vi "solar_read SOLARAppInfo.vi"(8 "error in (no error)":errorcluster, 11 "solar in":refnum<class "solar.lvclass">) -> (0 "error out":errorcluster, 2 "AppInfo":T1, 3 "solar out":refnum<class "solar.lvclass">)   [LabVIEW 2018, in "solar.lvclass"]
doc: "This returns the application information including application directories and versions information."
uses:
  solar.lvclass
  app/solar_app_ctl Info.ctl
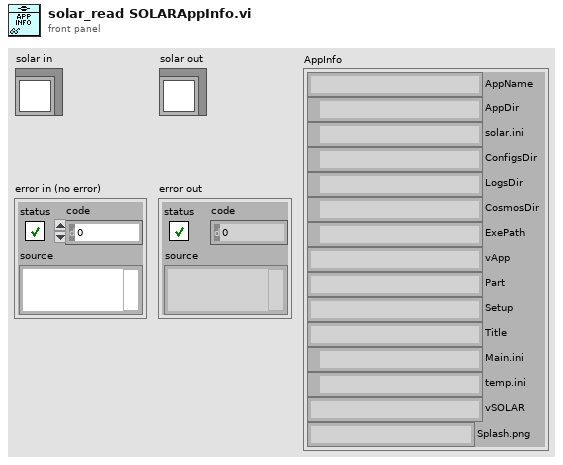
[diagram p1: front panel]
types:
  T1 = typedef "solar_app_ctl Info.ctl" = cluster{"AppName":string, "AppDir":path, "solar.ini":path, "ConfigsDir":path, "LogsDir":path, "CosmosDir":path, "ExePath":path, "vApp":string, "Part":string, "Setup":string, "Title":string, "Main.ini":path, "temp.ini":path, "vSOLAR":string, "Splash.png":string}
  T2 = typedef "solar_ctl SOLAR Refnum.ctl" = refnum<k1>
  T3 = typedef "solar_ctl SOLAR Global.ctl" = cluster{"Targets":T4[], "AppDir":path, "solar.ini":path, "ConfigsDir":path, "CosmosDir":path, "LogsDir":path, "ExePath":path, "ExeVersion":string, "PartNum":string, "AppSetup":string, "Title":string, "Main.ini":path, "Temp.ini":path, "vSOLAR":string, "Splash.png":string, "SplashWait":i32, "SOLARUE":refnum<user-event>, "VoyagerRefnum":T5, "QTimerRefnum":T6}
  T4 = typedef "solar_ctl Target Global.ctl" = cluster{"Target":string, "Q":refnum<queue>, "UE":refnum<user-event>, "VI":refnum<vi>, "Menu":refnum<k9>, "Data":refnum<data-value>, "Attributes":variant}
  T5 = typedef "solar_voy_ctl Voyager Refnum.ctl" = refnum<k1>
  T6 = typedef "solar_qtimer_ctl Refnum.ctl" = refnum<k1>
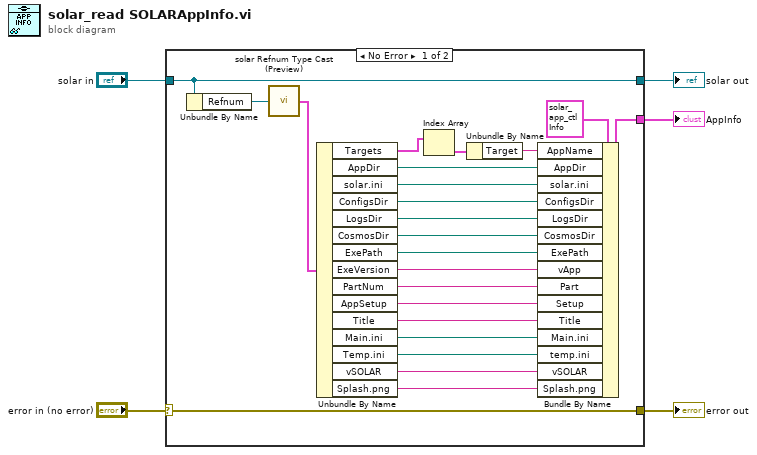
[diagram p0: block diagram]
diagram:
  n1 = case shown="No Error" "error in (no error)" {
    selector: "error in (no error)" -> [w26 w30]
    tunnel: "solar in" -> [w25 w29]
    tunnel: [w26 w30] -> w4
    tunnel: [w25 w29] -> w2
    tunnel: [w23 _] -> w1
    frame No Error {
      n2 = Unbundle By Name(w25) -> ("Refnum"=w28:T2)
      n3 = call "solar Refnum Type Cast (Preview).vi"("Refnum"=w28) -> ("SOLAR"=w27:T3)  [unwired: 8 in]
      n4 = Unbundle By Name(w27) -> ("Targets"=w22:T4[], "AppDir"=w19:path, "solar.ini"=w18:path, "ConfigsDir"=w17:path, "LogsDir"=w16:path, "CosmosDir"=w15:path, "ExePath"=w14:path, "ExeVersion"=w13:string, "PartNum"=w12:string, "AppSetup"=w11:string, "Title"=w10:string, "Main.ini"=w9:path, "Temp.ini"=w8:path, "vSOLAR"=w7:string, "Splash.png"=w6:string)
      n5 = Index Array(array=w22) -> (element=w21:T4)  [unwired: 1 in]
      n6 = Unbundle By Name(w21) -> ("Target"=w20:string)
      n7 = Bundle By Name(cluster=T1 {"AppName"="", "AppDir"=path "", "solar.ini"=path "", "ConfigsDir"=path "", "LogsDir"=path "", "CosmosDir"=path "", "ExePath"=path "", "vApp"="", "Part"="", "Setup"="", "Title"="", "Main.ini"=path "", "temp.ini"=path "", "vSOLAR"="", "Splash.png"=""} ("AppInfo"), "AppName"=w20, "AppDir"=w19, "solar.ini"=w18, "ConfigsDir"=w17, "LogsDir"=w16, "CosmosDir"=w15, "ExePath"=w14, "vApp"=w13, "Part"=w12, "Setup"=w11, "Title"=w10, "Main.ini"=w9, "temp.ini"=w8, "vSOLAR"=w7, "Splash.png"=w6) -> (w23:T1)
    }
    frame Error {
    }
  }
  "error out" <- w4
  "solar out" <- w2
  "AppInfo" <- w1
